vi "Do.vi"(8 "error in (no error)":errorcluster, 10 "Actor in":refnum<class "Actor.lvclass">, 11 "Set Control":refnum<class "Set Controls.lvclass">) -> (0 "error out":errorcluster, 2 "Actor out":refnum<class "Actor.lvclass">)   [LabVIEW 2014, in "tWorkerCommandRunner.lvlib" / "Set Controls.lvclass"]
doc: "(<B>Filename</B>: Actor Framework.lvlib:Message.lvclass:Do.vi)\n\nDefines what a message does when it is received by an actor. Generally, a message instructs an actor to invoke one of its methods. By default, this method does nothing. A child class must override it to define behavior. Create a child class by using the Actor Framework Message Maker dialog box."
uses:
  Set Controls.lvclass
  <vilib>/ActorFramework/Actor/Actor.lvclass
  tWorkerCommandRunner/tWorkerCommandRunner.lvclass
  Set Controls.lvclass/Set Controls.ctl
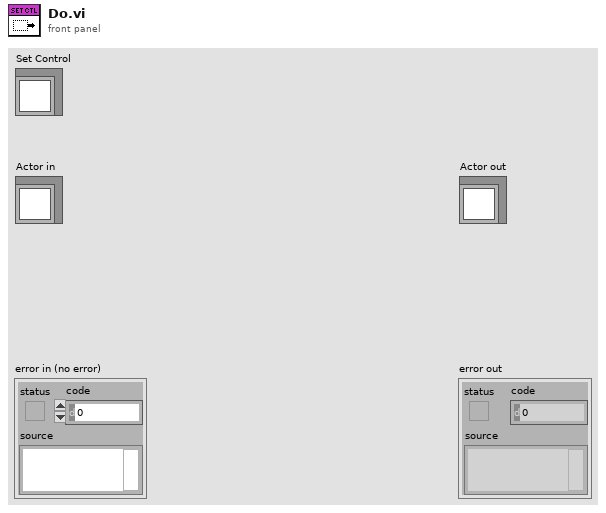
[diagram p1: front panel]
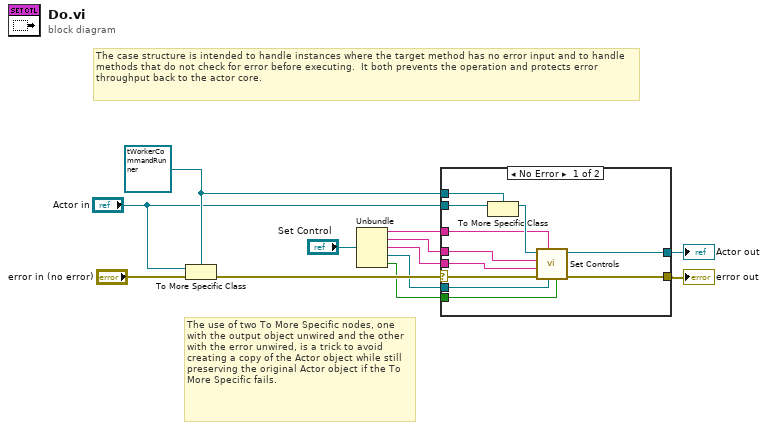
[diagram p0: block diagram]
diagram:
  w11 = refnum<class "tWorkerCommandRunner.lvclass"> refnum ("Actor in")
  # "The use of two To More Specific nodes, one with the output object unwired and the other with the error unwired, is a trick to avoid creating a copy of the Actor object while still preserving the original Actor object if the To More Specific fails."
  # "The case structure is intended to handle instances where the target method has no error input and to handle methods that do not check for error before executing.  It both prevents the operation and protects error throughput back to the actor core."
  n1 = To More Specific Class(target class=w11, reference="Actor in", error in="error in (no error)") -> (error out=w12:errorcluster)  [unwired: 1 out]
  n2 = Unbundle("Set Control") -> (w10:string, w9:string, w8:string, w7:refnum<class "tBSONDocument.lvclass">, w1:bool)
  n3 = case shown="No Error" w12 {
    selector: w12 -> [w19 w25]
    tunnel: [w18 w25] -> w6
    tunnel: [w20 w24] -> w5
    tunnel: "Actor in" -> [w23 w24]
    tunnel: w11 -> [w22 _]
    tunnel: w10 -> [w17 _]
    tunnel: w9 -> [w14 _]
    tunnel: w8 -> [w16 _]
    tunnel: w7 -> [w15 _]
    tunnel: w1 -> [w13 _]
    frame No Error {
      n4 = To More Specific Class(target class=w22, reference=w23) -> (specific class reference=w21:refnum<class "tWorkerCommandRunner.lvclass">)  [unwired: 1 in, 1 out]
      n5 = call "Set Controls.vi"("Ignore Non-existing Controls"=w13, "VI Control Values"=w15, "Project Path"=w17, "error in (no error)"=w19, "VI Path"=w16, "Target Name"=w14, "tWorkerCommandRunner in"=w21) -> ("error out"=w18:errorcluster, "tWorkerCommandRunner out"=w20:refnum<class "tWorkerCommandRunner.lvclass">)  [unwired: 3 in]
    }
    frame Error {
      # "If type check fails, pass the original object out again."
    }
  }
  "error out" <- w6
  "Actor out" <- w5
